vi "To Global Coordinates.vi"(8 "error in":errorcluster, 10 "Center/Orientation":T1, 11 "Local Coordinates":refnum<class "Vec3d.lvclass">) -> (0 "error out":errorcluster, 3 "Global Coordinates":refnum<class "Vec3d.lvclass">)   [LabVIEW 2023]
uses:
  Type Definitions/Position_Orientation.ctl
  Vec3d Class/Vec3d.lvclass
  Orient3d Class/Orient3d.lvclass
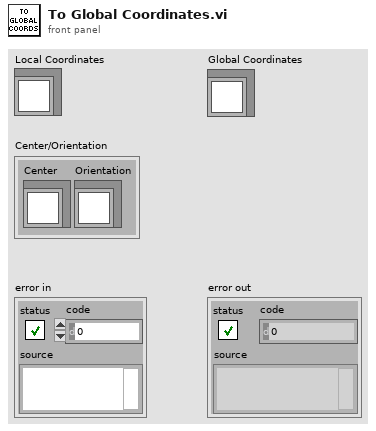
[diagram p1: front panel]
types:
  T1 = typedef "Position_Orientation.ctl" = cluster{"Center":refnum<class "Vec3d.lvclass">, "Orientation":refnum<class "Orient3d.lvclass">}
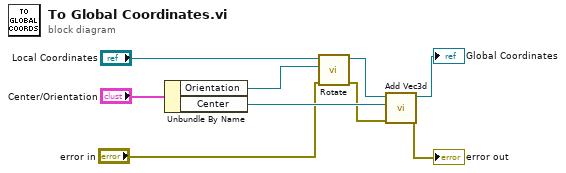
[diagram p0: block diagram]
diagram:
  n1 = Unbundle By Name("Center/Orientation") -> ("Orientation"=w7:refnum<class "Orient3d.lvclass">, "Center"=w6:refnum<class "Vec3d.lvclass">)
  n2 = call-dynamic "Rotate.vi"("error in"="error in", "Orient3d in"=w7, "Vec3d in"="Local Coordinates") -> ("error out"=w4:errorcluster, "Vec3d out"=w1:refnum<class "Vec3d.lvclass">)  [unwired: 7 in]
  n3 = call-dynamic "Add Vec3d.vi"("error in (no error)"=w4, 10:"Vec3d Class in"=w6, 11:"Vec3d Class in"=w1) -> ("error out"=→"error out":errorcluster, "Vec3d Class out"=→"Global Coordinates":refnum<class "Vec3d.lvclass">)  [unwired: 7 in]
